vi "1-4040_SetSampleDelayTime.vi"(8 "Error in":errorcluster caption="Error In", 10 "Sample Delay Time(ms)":i32, 11 "Visa IO":refnum<visa-resource-name>) -> (0 "error out":errorcluster, 3 "SetSuccessful?":bool)   [LabVIEW 2017]
uses:
  <vilib>/Instr/_visa.llb/VISA Flush IO Buffer Mask.ctl
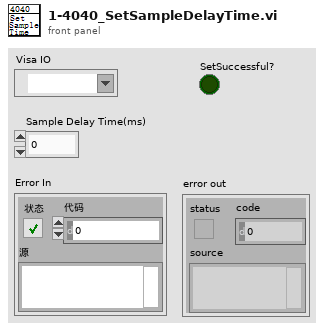
[diagram p1: front panel]
types:
  T1 = typedef "VISA Flush IO Buffer Mask.ctl" = u16
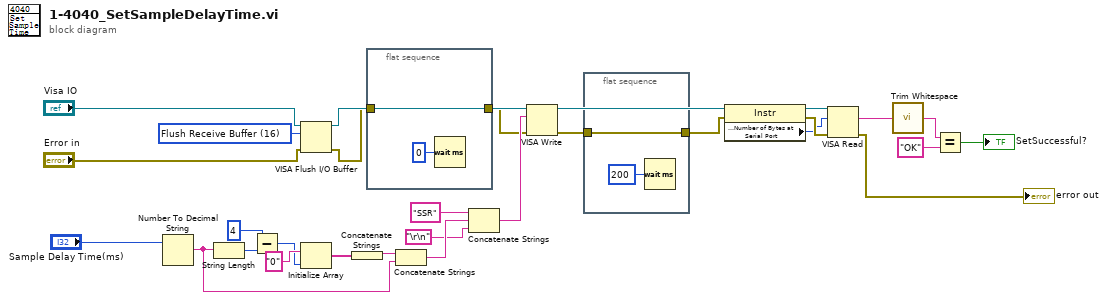
[diagram p0: block diagram]
diagram:
  w7 = T1 16 items=["Flush Receive Buffer"=16, "Write Transmit Buffer to Device"=32, "Flush Receive Buffer (No I/O)"=64, "Flush Transmit Buffer"=128] ("Mask")
  n1 = Number To Decimal String(number="Sample Delay Time(ms)") -> (decimal integer string=w22:string)  [unwired: 1 in]
  n2 = String Length(string=w22) -> (length=w16:i32)
  n3 = Subtract(x=4, y=w16) -> (x-y=w18:i32)
  n4 = VISA Flush I/O Buffer(VISA resource name="Visa IO", mask (16)=w7, error in (no error)="Error in") -> (VISA resource name out=w5:refnum<visa-resource-name>, error out=w3:errorcluster)
  n5 = Initialize Array("0", w18) -> (w20:string[])
  n6 = Concatenate Strings(w20) -> (w21:string)
  n7 = flat-sequence {
    tunnel: w3 -> [w30]
    tunnel: [w30] -> w2
    frame #0 {
      n8 = Wait (ms)(milliseconds to wait=u32 0) -> ()  [unwired: 1 out]
    }
  }
  n9 = Concatenate Strings(w21, w22) -> (w23:string)
  n10 = Concatenate Strings("SSR" ("写入缓冲区"), w23, "\r\n") -> (w24:string)
  n11 = VISA Write(VISA resource name=w5, write buffer=w24, error in (no error)=w2) -> (VISA resource name out=w28:refnum<visa-resource-name>, error out=w12:errorcluster)  [unwired: 1 out]
  n12 = flat-sequence {
    tunnel: w12 -> [w32]
    tunnel: [w32] -> w11
    frame #0 {
      n13 = Wait (ms)(milliseconds to wait=u32 200) -> ()  [unwired: 1 out]
    }
  }
  n14 = property class="Instr"(reference=w28, error in=w11) -> (reference out=w27:refnum<visa-resource-name>, error out=w26:errorcluster, "Serial Settings:Number of Bytes at Serial Port"=w25:u32)
  n15 = VISA Read(VISA resource name=w27, byte count=w25, error in (no error)=w26) -> (read buffer=w29:string, error out=→"error out":errorcluster)  [unwired: 2 out]
  n16 = call <vilib>:"Trim Whitespace.vi"("string"=w29) -> ("trimmed string"=w10:string)  [unwired: 1 in]
  n17 = Equal?(x=w10, y="OK") -> (x = y?=→"SetSuccessful?":bool)
